vi "test.vi"() -> ()   [LabVIEW 2017]
uses:
  <instrlib>/niUSRP/niUSRP Fetch Rx Data (CDB WDT).vi
  <vilib>/measure/maspectr.llb/FFT Power Spectrum and PSD for 1 Chan (CDB).vi
  <vilib>/measure/NI_MAPro.lvlib
panel:
  out "PSC  convolution":dbl[](graph)
  out "CPICH convolution":dbl[](graph)
  out "IQ Graph":cdb[](graph) caption="CCPCH channel dibits"
  out "dibits energy":dbl[][](graph)
  in  "Data":cdb[](array[numeric])=array[200000 elements]
  in  "averaging parameters":T1={"averaging mode"=enum."RMS averaging", "weighting mode"=enum."Exponential", "number of averages"=50} {"number of averages" min=1}
  out "Waveform Graph":cluster{"f0":dbl, "df":dbl, "magnitude":dbl[]}(graph)
  in  "IQ rate":dbl=7680000.0 format="%#_13p"
  in  "gain":dbl=60.0 format="%#_6f"
  in  "device name":refnum<k15>="MyB210"
  in  "freq.":dbl=2137400000.0 format="%#_6p"
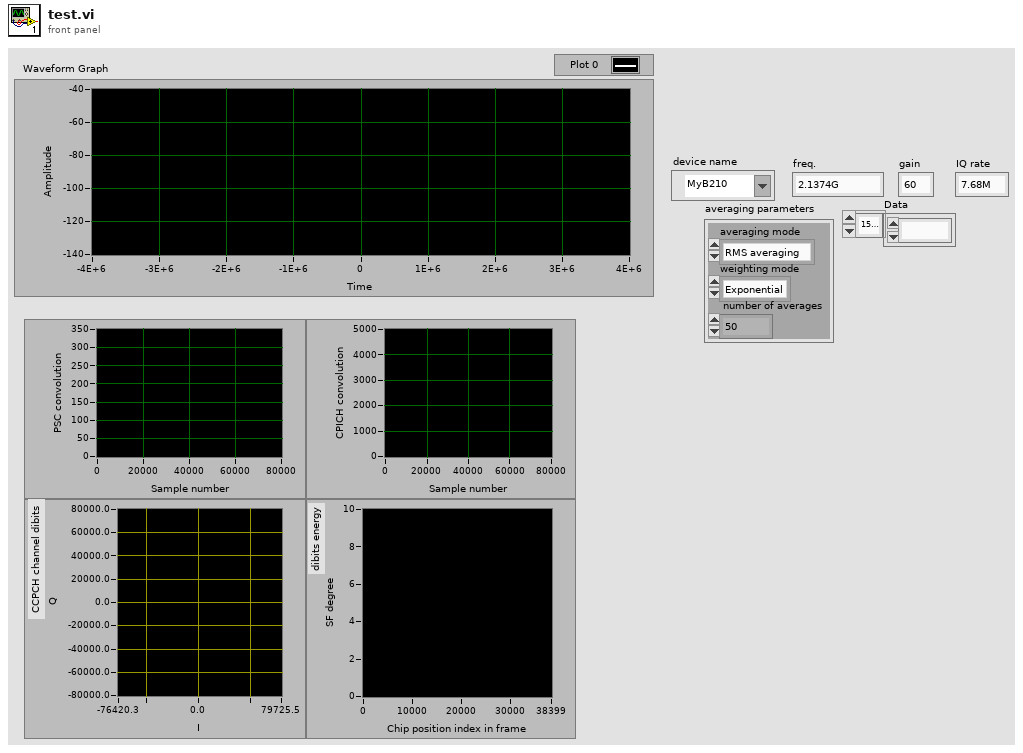
[diagram p1: front panel]
types:
  T1 = cluster{"averaging mode":enum16{"No averaging", "Vector averaging", "RMS averaging", "Peak hold"}, "weighting mode":enum16{"Linear", "Exponential"}, "number of averages":u32}
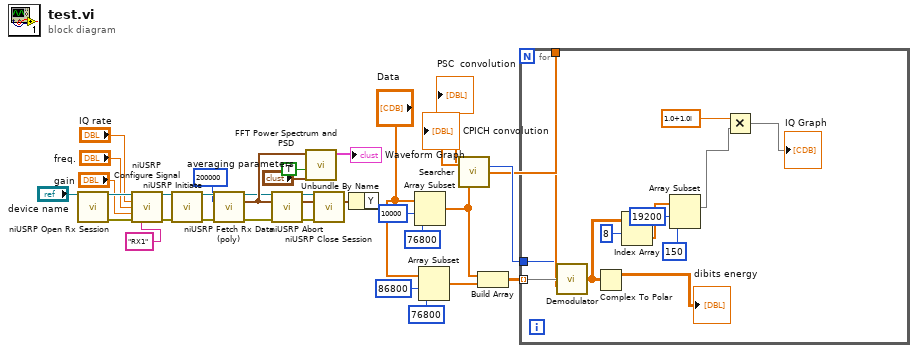
[diagram p0: block diagram]
diagram:
  n1 = call <instrlib>:"niUSRP Open Rx Session.vi"("device names"="device name") -> ("session handle out"=w29:refnum<k15>, "error out"=w28:errorcluster)  [unwired: 13 in]
  n2 = call <instrlib>:"niUSRP Configure Signal.vi"("session handle"=w29, "IQ rate"="IQ rate", "carrier frequency"="freq.", "gain"="gain", "error in (no error)"=w28, "active antenna"="RX1") -> ("session handle out"=w20:refnum<k15>, "error out"=w21:errorcluster)  [unwired: 5 in, 3 out]
  n3 = call <instrlib>:"niUSRP Initiate.vi"("session handle"=w20, "error in (no error)"=w21) -> ("session handle out"=w22:refnum<k15>, "error out"=w23:errorcluster)  [unwired: 12 in]
  n4 = call-poly <instrlib>:"niUSRP Fetch Rx Data (poly).vi"("session handle"=w22, "number of samples"=200000 ("channel 2"), "error in (no error)"=w23) -> ("session handle out"=w27:refnum<k15>, "data"=w31:waveform(cdb), "error out"=w25:errorcluster)  [unwired: 9 in, 1 out]
  n5 = call <instrlib>:"niUSRP Abort.vi"("session handle"=w27, "error in (no error)"=w25) -> ("session handle out"=w24:refnum<k15>, "error out"=w26:errorcluster)  [unwired: 12 in]
  n6 = call-poly <vilib>:"FFT Power Spectrum and PSD.vi"("averaging parameters"="averaging parameters", "dB On (F)"=TRUE, "time signal"=w31) -> ("Power Spectrum / PSD"=→"Waveform Graph":cluster{"f0":dbl, "df":dbl, "magnitude":dbl[]})  [unwired: 5 in, 3 out]
  n7 = call <instrlib>:"niUSRP Close Session.vi"("session handle"=w24, "error in (no error)"=w26) -> ()  [unwired: 13 in, 1 out]
  n8 = Unbundle By Name(w31) -> ()  [unwired: 1 out]
  n9 = Array Subset(array="Data", index=10000, length=76800) -> (w5:cdb[])
  n10 = Array Subset(array="Data", index=86800, length=76800) -> (w7:cdb[])
  n11 = call "Searcher.vi"("сегмент сигнала\nс SDR-приемника"=w5) -> ("CPICH convolution"=→"CPICH convolution":dbl[], "PSC  convolution"=→"PSC  convolution":dbl[], "l est"=w4:i32, "I"=w3:cdb[])  [unwired: 11 in]
  n12 = Build Array(w5, w7) -> (w6:cdb[][])
  n13 = for {
    tunnel: w6 -> [w44] mode=indexing
    tunnel: w3 -> [w43]
    tunnel: w4 -> [w42]
    n14 = call "Demodulator.vi"("Initial df"=w42, "rx"=w44, "I"=w43) -> ("all symbols"=w41:cdb[][])  [unwired: 12 in]
    n15 = Complex To Polar(r * e^(i*theta)=w41) -> (r=→"dibits energy":dbl[][])  [unwired: 1 out]
    n16 = Index Array(array=w41, index (row)=8) -> (element=w39:cdb[])  [unwired: 1 in]
    n17 = Array Subset(array=w39, index=19200, length=150) -> (w35:cdb[])
    n18 = Multiply(x=cdb 1.0+1.0i, y=w35) -> (x*y=→"IQ Graph":cdb[])
  }
